vi "Create NI 9482 - Digital Output.vi"(8 "error in":errorcluster, 11 "channel settings":T1[](array[typedef])) -> (0 "error out":errorcluster, 3 "NI 9482 out":refnum<class "NI 9482.lvclass">)   [LabVIEW 2017, in "Scan Engine Scripting.lvlib" / "NI 9482.lvclass"]
doc: "Creates and configures an instance of a 9482 module that can be used to set a slot in a scan engine custom device chassis."
uses:
  NI 9482.lvclass
  Mode Classes/Controls/digital channel settings.ctl
  Mode Classes/Digital Output Mode/Digital Output Mode.lvclass
  C:/dev/niveristand-scan-engine-ethercat-custom-device/Custom Device Source/Scripting/Modules/Mode Classes/Mode/Mode.lvclass
  12362a5c-7dcd-4795-9f7c-dc2dd115e12c.vi
  Scan Engine Scripting.lvlib
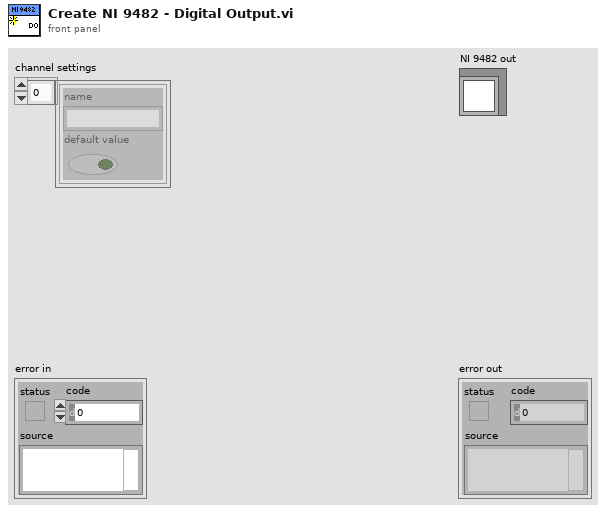
[diagram p1: front panel]
types:
  T1 = typedef "Scan Engine Scripting.lvlib/digital channel settings.ctl" = cluster{"name":string, "default value":bool}
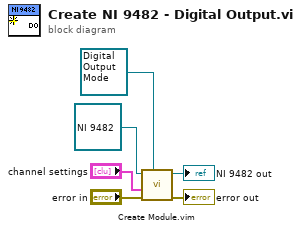
[diagram p0: block diagram]
diagram:
  n1 = call "Create Module.vim"("mode in"=refnum<class "Digital Output Mode.lvclass"> refnum ("Scan Engine Scripting.lvlib:Digital Output Mode.lvclass"), "error in"="error in", "channel settings"="channel settings", "module in"=refnum<class "NI 9482.lvclass"> refnum ("NI 9482 out")) -> ("error out"=→"error out":errorcluster, "module out"=→"NI 9482 out":refnum<class "NI 9482.lvclass">)  [unwired: 6 in]
